vi "String Fomula In.vi"(8 "error in":errorcluster, 10 "formula":string, 11 "Alicat_P in":refnum<class "P.lvclass">) -> (0 "error out":errorcluster, 3 "Alicat_P out":refnum<class "P.lvclass">)   [LabVIEW 2013, in "Alicat.lvlib" / "P.lvclass"]
uses:
  P.lvclass
  P.lvclass/P.ctl
  <vilib>/gmath/NI_Gmath.lvlib
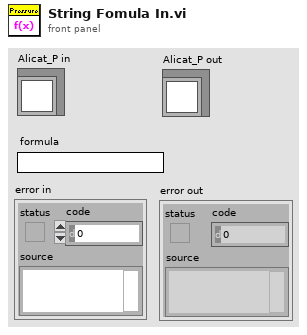
[diagram p1: front panel]
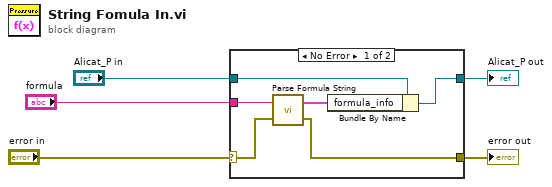
[diagram p0: block diagram]
diagram:
  n1 = case shown="No Error" "error in" {
    selector: "error in" -> [w7 w13]
    tunnel: [w6 w13] -> w4
    tunnel: [w8 w12] -> w2
    tunnel: "Alicat_P in" -> [w10 w12]
    tunnel: "formula" -> [w11 _]
    frame No Error {
      n2 = call <vilib>:"Parse Formula String.vi"("error in (no error)"=w7, "formula"=w11) -> ("error out"=w6:errorcluster, "Parsed Formula"=w9:cluster{"Table":i32[][], "Y Values":dbl[]})
      n3 = Bundle By Name(cluster=w10, "formula_info"=w9) -> (w8:refnum<class "P.lvclass">)
    }
    frame Error {
    }
  }
  "error out" <- w4
  "Alicat_P out" <- w2
